vi "PXIe-4139 Updated Channels (RT).vi"(5 "Channel Type":T1 items=["Voltage Controlled", "Current Controlled"], 7 "Channel":string, 8 "error in (no error)":errorcluster, 9 "FIFO Indexes":i32[](array[numeric]), 10 "Data In":dbl[](array[numeric]), 11 "resource name In":refnum<k15>) -> (0 "error out":errorcluster, 2 "Data Out":dbl[](array[numeric]), 3 "resource name Out":refnum<k15>)   [LabVIEW 2023, in "PXIe-4139 Custom Device.lvlib"]
uses:
  PXIe-4139 Custom Device.lvlib
  Controls/Channel Type.ctl
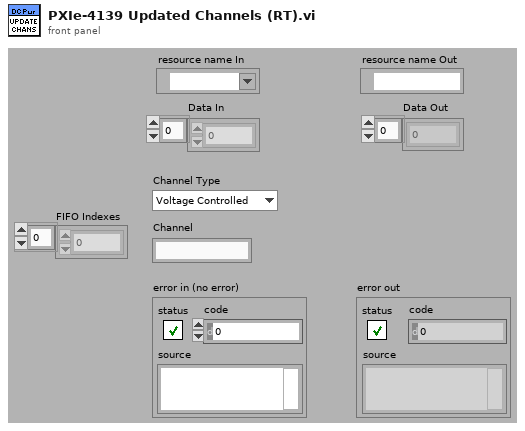
[diagram p1: front panel]
types:
  T1 = typedef "PXIe-4139 Custom Device.lvlib/Channel Type.ctl" = i32
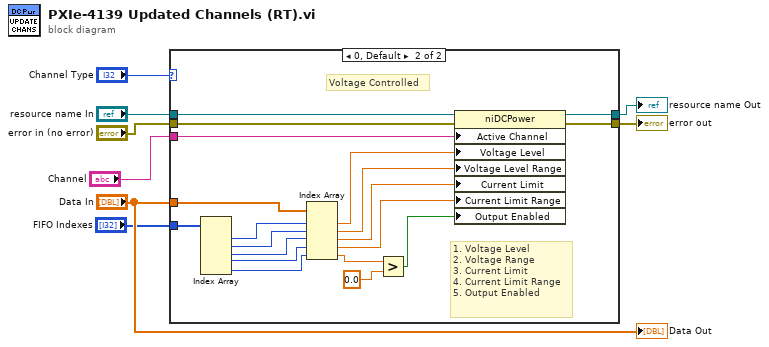
[diagram p0: block diagram]
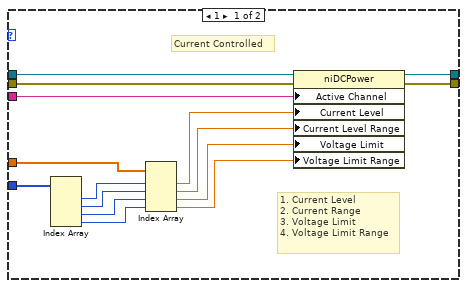
[diagram p2: hidden frame]
diagram:
  n1 = case shown="0, Default" "Channel Type" {
    tunnel: "resource name In" -> [w23 w42]
    tunnel: "Data In" -> [w22 w41]
    tunnel: [w18 w37] -> w6
    tunnel: [w17 w36] -> w7
    tunnel: "error in (no error)" -> [w16 w35]
    tunnel: "Channel" -> [w14 w33]
    tunnel: "FIFO Indexes" -> [w13 w32]
    frame 1 {
      # "1. Current Level\n2. Current Range\n3. Voltage Limit\n4. Voltage Limit Range"
      # "Current Controlled"
      n2 = Index Array(array=w13) -> (element #1=w12:i32, element #2=w11:i32, element #3=w10:i32, element #4=w9:i32)  [unwired: 4 in]
      n3 = Index Array(array=w22, index #1=w12, index #2=w11, index #3=w10, index #4=w9) -> (element #1=w15:dbl, element #2=w21:dbl, element #3=w20:dbl, element #4=w19:dbl)
      n4 = property class="niDCPower"(reference=w23, error in=w16, "Active Channel"=w14, "Current Level"=w15, "Current Level Range"=w21, "Voltage Limit"=w20, "Voltage Limit Range"=w19) -> (reference out=w18:refnum<k15>, error out=w17:errorcluster)
    }
    frame 0, Default {
      # "1. Voltage Level\n2. Voltage Range\n3. Current Limit\n4. Current Limit Range\n5. Output Enabled"
      # "Voltage Controlled"
      n5 = Index Array(array=w32) -> (element #1=w31:i32, element #2=w30:i32, element #3=w29:i32, element #4=w28:i32, element #5=w27:i32)  [unwired: 5 in]
      n6 = Index Array(array=w41, index #1=w31, index #2=w30, index #3=w29, index #4=w28, index #5=w27) -> (element #1=w34:dbl, element #2=w40:dbl, element #3=w39:dbl, element #4=w38:dbl, element #5=w26:dbl)
      n7 = Greater?(x=w26, y=0.0) -> (0:w24:bool)
      n8 = property class="niDCPower"(reference=w42, error in=w35, "Active Channel"=w33, "Voltage Level"=w34, "Voltage Level Range"=w40, "Current Limit"=w39, "Current Limit Range"=w38, "Output Enabled"=w24) -> (reference out=w37:refnum<k15>, error out=w36:errorcluster)
    }
  }
  "resource name Out" <- w6
  "error out" <- w7
  "Data Out" <- "Data In"
